vi "Launch Target Actor.vi"() -> ()   [LabVIEW 2023]
uses:
  MSS Target Actor/MSS Target Actor.lvclass
  Thermometer/Thermometer DAQmx RTD Cont CFG/Thermometer DAQmx RTD Cont CFG.lvclass
  DIO/DO DAQmx Fixed Freq PWM CFG/DO DAQmx Fixed Freq PWM CFG.lvclass
  DIO/Virtual DIO/Virt PWM Fixed Freq Generator/Virt DAQmx Fixed Freq PWM Generator.lvclass
  AI/AI Cont CFG/AI DAQmx Cont CFG.lvclass
  AI/AI Simulated CFGs/AI DAQmx Cont CFG Simulated.lvclass
  Tests/No Op DAQmx Instrument/DAQmx No Op.lvclass
  gitlab/imponator-series-actor/Imponator Series Actor/Virt Instrs/4-20mA 0-100/Virt Convert 4-20mA 0-100.lvclass
  MSS Target Actor/MSS Target Actor.lvclass/MSS Target Actor.ctl
  <vilib>/ni/Actors/Network Endpoint Actors/Protocols/Network Stream Strategy/Netowrk Stream Listener/Network Stream Listener.lvclass
  <vilib>/ActorFramework/Actor/Actor.lvclass
  gitlab/imponator-series-actor/Imponator Series Actor/Virt Instrs/4-20mA -40-60/Virt Convert 4-20mA -40-60C.lvclass
panel:
  in  "error in":errorcluster
  out "error out":errorcluster
  # "Target"
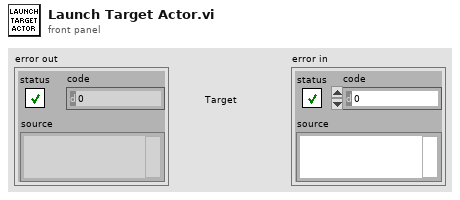
[diagram p1: front panel]
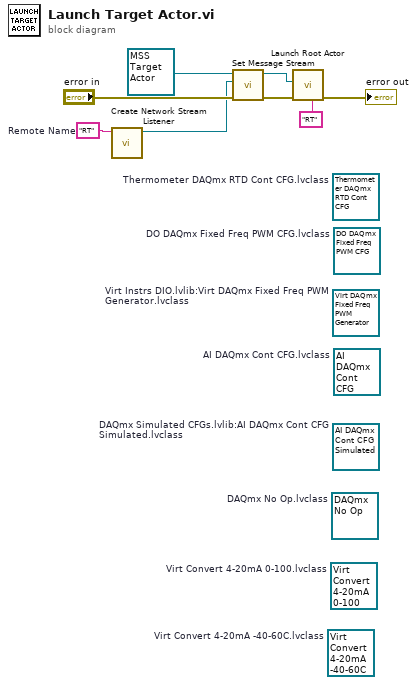
[diagram p0: block diagram]
diagram:
  (unwired) refnum<class "Virt Convert 4-20mA -40-60C.lvclass"> refnum  # Virt Convert 4-20mA -40-60C.lvclass
  (unwired) refnum<class "Virt Convert 4-20mA 0-100.lvclass"> refnum  # Virt Convert 4-20mA 0-100.lvclass
  (unwired) refnum<class "DAQmx No Op.lvclass"> refnum  # DAQmx No Op.lvclass
  (unwired) refnum<class "AI DAQmx Cont CFG Simulated.lvclass"> refnum  # DAQmx Simulated CFGs.lvlib:AI DAQmx Cont CFG Simulated.lvclass
  (unwired) refnum<class "AI DAQmx Cont CFG.lvclass"> refnum  # AI DAQmx Cont CFG.lvclass
  (unwired) refnum<class "Virt DAQmx Fixed Freq PWM Generator.lvclass"> refnum  # Virt Instrs DIO.lvlib:Virt DAQmx Fixed Freq PWM Generator.lvclass
  (unwired) refnum<class "DO DAQmx Fixed Freq PWM CFG.lvclass"> refnum  # DO DAQmx Fixed Freq PWM CFG.lvclass
  (unwired) refnum<class "Thermometer DAQmx RTD Cont CFG.lvclass"> refnum  # Thermometer DAQmx RTD Cont CFG.lvclass
  w7 = "RT"  # Remote Name
  n1 = call <vilib>:"Create Network Stream Listener.vi"("Name"=w7) -> ("Network Stream Listener"=w1:refnum<class "Network Stream Listener.lvclass">)  [unwired: 10 in]
  n2 = call "Set Message Stream.vi"("Message Stream.lvclass"=w1, "CRIO MSS Test Actor in"=refnum<class "MSS Target Actor.lvclass"> refnum ("MSS Target Actor.lvlib:MSS Target Actor.lvclass")) -> ("CRIO MSS Test Actor out"=w6:refnum<class "MSS Target Actor.lvclass">)  [unwired: 9 in]
  n3 = call <vilib>:"Launch Root Actor.vi"("Debug Alias"="RT", "error in (no error)"="error in", "Actor"=w6) -> ("error out"=→"error out":errorcluster)  [unwired: 7 in, 1 out]
